vi "Streamlined FPGA.vi"() -> ()   [LabVIEW 2009]
uses:
  <vilib>/eio/EIONode/EIONode.xnode
  <vilib>/rvi/eio/nirviEIOImplementation/nirviEIOImplementation.xnode
  <vilib>/rvi/eio/common/nirviEmuTemplateMethod_noerrors.vi
  <vilib>/rvi/eio/common/nirviEmuClasses.ctl
  Instance           3 24Saved   Streamlined FPGA .vi
  Instance           4 24Saved   Streamlined FPGA .vi
  Instance           5 24Saved   Streamlined FPGA .vi
  Instance           2 24Saved   Streamlined FPGA .vi
  <vilib>/rvi/DataTransferAndStorage/Container/XNode/niFpgaContainer.xnode
  <vilib>/rvi/interface/RandomDataEmulation/niFpgaRandomDataHandleErrors.vi
  <vilib>/rvi/interface/RandomDataEmulation/nirviRandomDataFPGAFIFO.vi
  <vilib>/rvi/DataTransferAndStorage/Container/Common/niFpgaContainerMethod.ctl
  <vilib>/rvi/DataTransferAndStorage/Container/Common/niFpgaTransferTypeControl.ctl
panel:
  in  "smooth":bool
  out ">= x":bool
  out ">= y":bool
  out "xmax":i32
  out "xval":i32
  out "xmin":i32
  out ">=":bool
  in  "Rec2 Ymin":i32
  in  "Rec2 Xmin":i32
  in  "Rec1 Ymin":i32
  in  "Rec1 Xmin":i32
  in  "Rec2 Ymax":i32
  in  "Rec1 Ymax":i32
  in  "Rec2 Xmax":i32
  in  "Rec1 Xmax":i32
  out "sort!":bool
  in  "Maximum Width":i16
  in  "Maximum Height":i16
  in  "trigger on all":bool
  out "sort pulse":i16
  in  "Baselines":i16[](array[numeric])=[0, 0, 0, 0]
  in  "Sb":i8(ring)=1 items=["PMT1", "PMT2", "PMT3", "PMT4"]
  in  "Sa":i8(ring) items=["PMT1", "PMT2", "PMT3", "PMT4"]
  in  "Sort Case":i8(ring)=1 items=["FP", "Magnitude"]
  out "Full 2":bool
  in  "sort?":bool
  out "Drop counter":u32
  out "sort counter":u32
  in  "PMT to detect drops on":u8
  in  "Minimum Height":i16
  in  "Minimum Width":i16
  in  "Ticks between acquires (Ticks)":u32=200
  in  "Gain 1":i16(slide) scale=-32767.0..32767.0
  in  "Gain 2":i16(slide) scale=-32767.0..32767.0
  in  "Gain 3":i16(slide) scale=-32767.0..32767.0
  in  "Gain 4":i16(slide) scale=-32767.0..32767.0
  in  "amplitude":i16
  in  "1/Frequency \n(ticks)":u32
  in  "Burst \nCycles":i32
  in  "delay [us]":u32=20 min=1 max=8000
  # "Acquisition and Detection"
  # "FP and Sorting Parameters"
  # "Sorting Pulse\nGenerator"
  # "Events"
  # "PMT Controls"
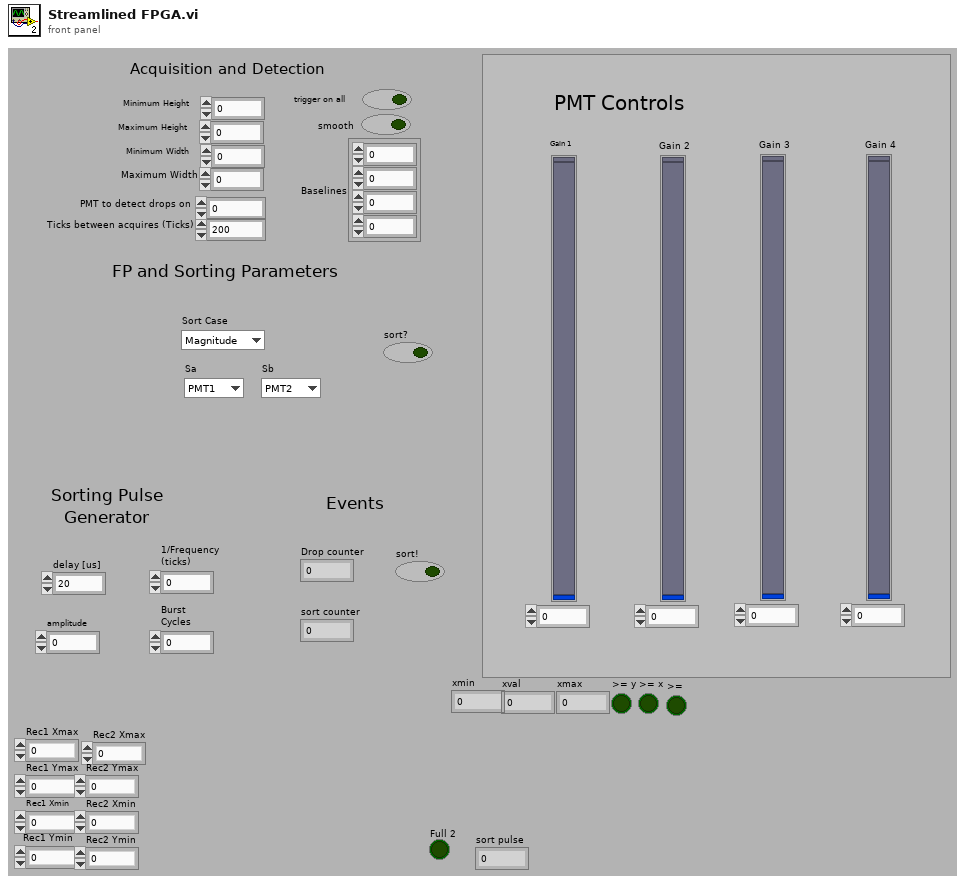
[diagram p1: front panel]
types:
  T1 = typedef "nirviEmuClasses.ctl" = enum16{"IO Read", "IO Write", "Method", "Property Read", "Property Write"}
  T2 = typedef "niFpgaContainerMethod.ctl" = enum16{"Write", "Read", "Clear", "Get Number of Elements to Write", "Get Number of Elements to Read", "Enable", "Disable", "Flush and Disable", "Get Stream State"}
  T3 = typedef "niFpgaTransferTypeControl.ctl" = enum16{"Target-Scoped", "Host to Target - DMA", "Target to Host - DMA", "Peer to Peer Reader", "Peer to Peer Writer", "Bidirectional"}
  T4 = cluster{"Rec1 Xmax":i32, "Rec1 Ymax":i32, "Rec1 Xmin":i32, "Rec1 Ymin":i32, "Rec2 Xmax":i32, "Rec2 Ymax":i32, "Rec2 Xmin":i32, "Rec2 Ymin":i32}
  T5 = cluster{bool, "max":i16[], "sum":i32[], "time inside":i32, "time outside":i32, "timeoutside-1":i32}
  T6 = cluster{"maxes":i16[], "sums":i32[], "time inside":i32, "time outside":i32}
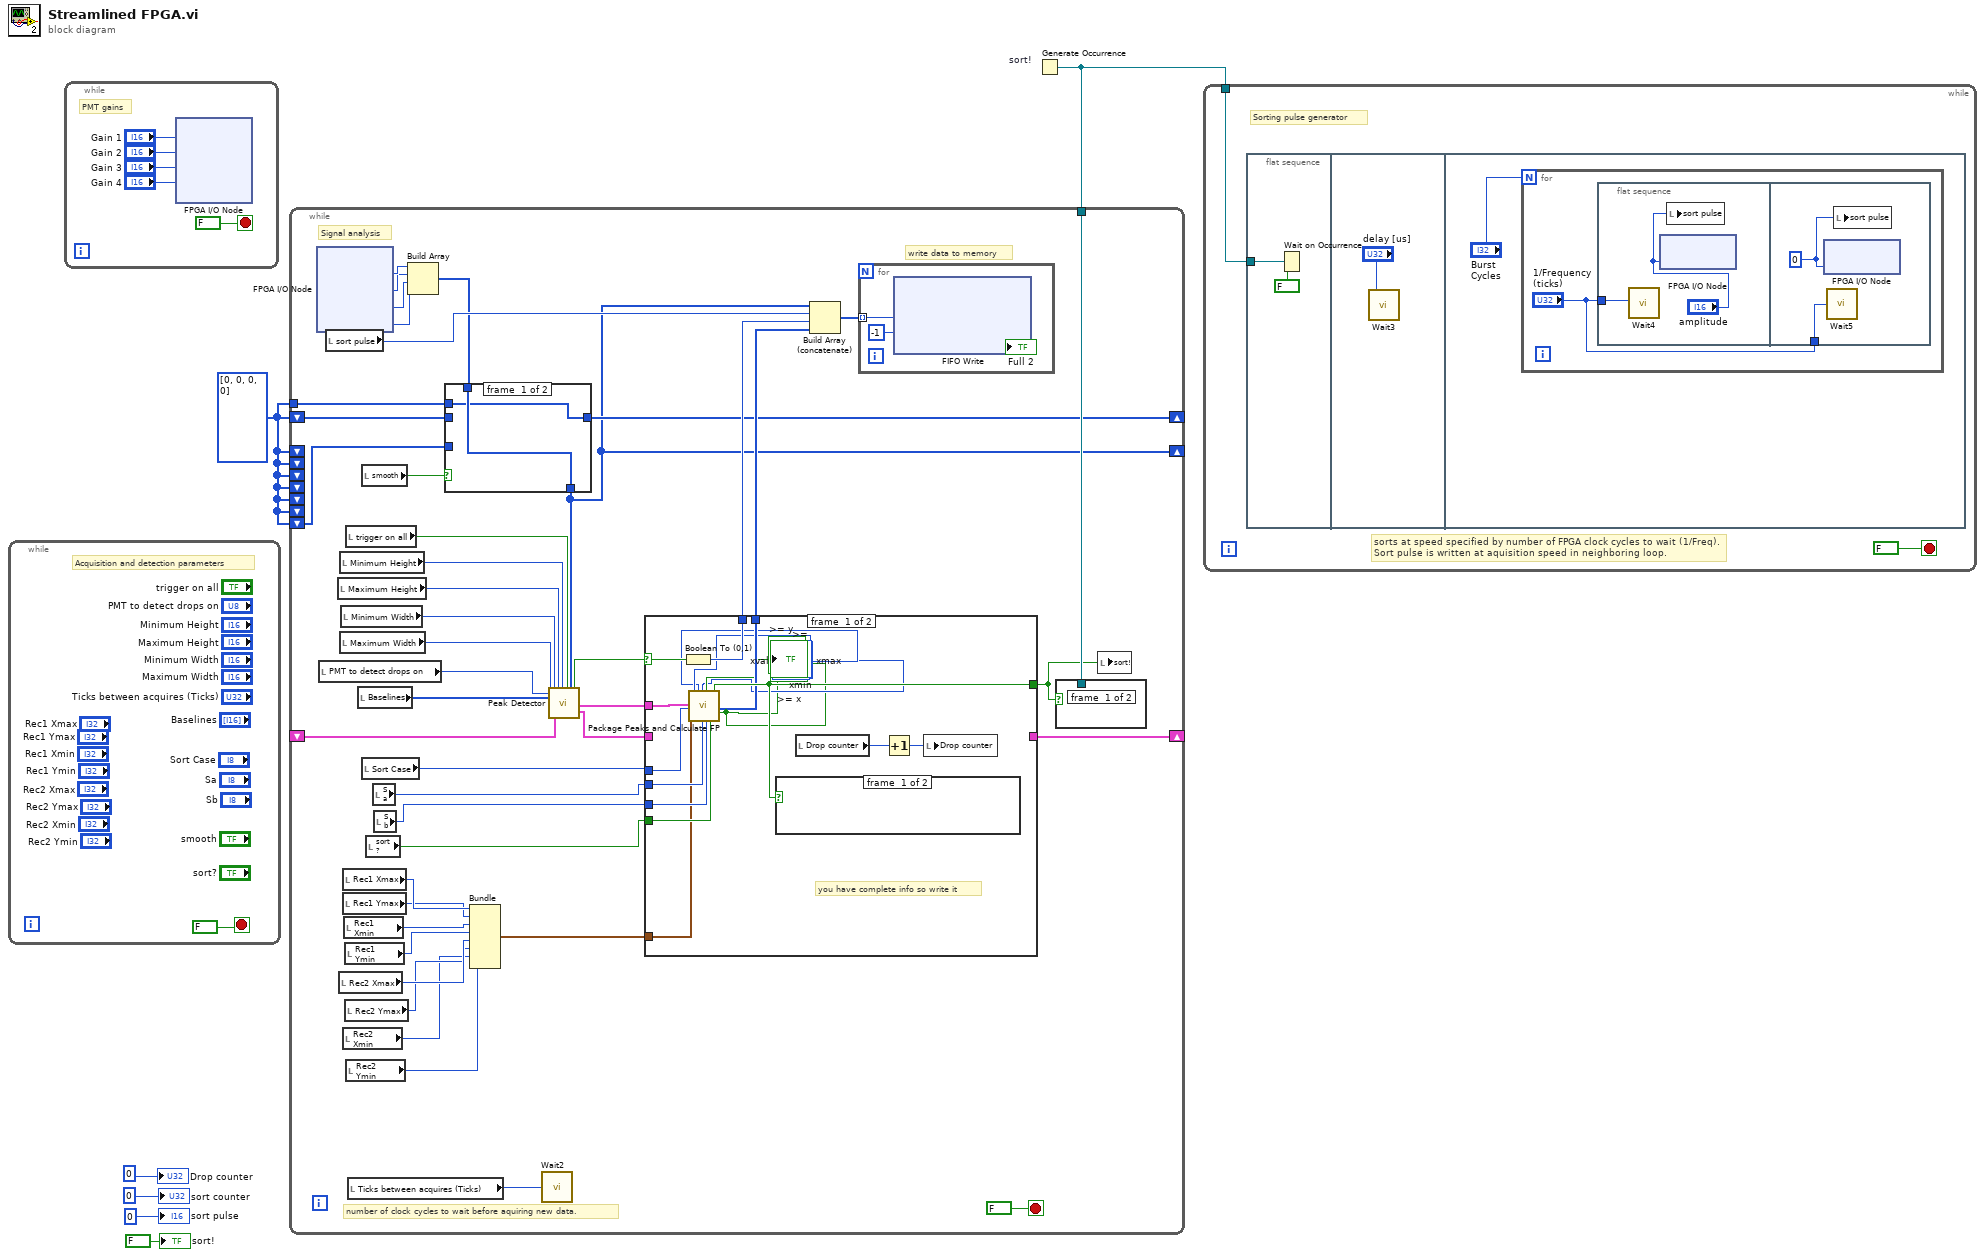
[diagram p0: block diagram]
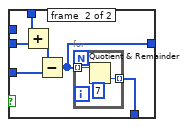
[diagram p2: hidden frame]
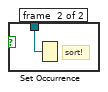
[diagram p3: hidden frame]
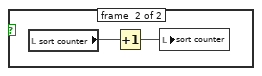
[diagram p4: hidden frame]
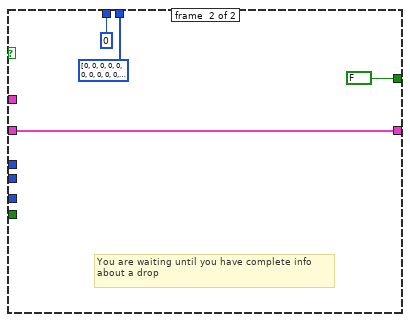
[diagram p5: hidden frame]
diagram:
  w1 = i32[] [0, 0, 0, 0] ("appended array")
  n1 = while {
    stop <- FALSE stop-if-true
    # "Acquisition and detection parameters"
  }
  n2 = while {
    stop <- FALSE stop-if-true
    # "PMT gains"
    n3 = xnode "FPGA I/O Node"("AO0"="Gain 1", "AO1"="Gain 2", "AO2"="Gain 3", "AO3"="Gain 4") -> ()  [unwired: 4 in, 4 out]
  }
  n4 = Generate Occurrence "sort!"() -> (w6:refnum<k4>)
  n5 = while {
    shift-right: [w99] -> _
    shift-left: _ -> [w86]
    tunnel: w6 -> [w84]
    shift-right: [w59] -> _
    shift-left: w1 -> [w63]
    shift-right: [w58] -> _
    shift-left: w1 -> [_]
    shift-left: w1 -> [_]
    shift-left: w1 -> [_]
    shift-left: w1 -> [_]
    shift-left: w1 -> [_]
    shift-left: w1 -> [_]
    shift-left: w1 -> [w62]
    tunnel: w1 -> [w61]
    stop <- FALSE stop-if-true
    # "number of clock cycles to wait before aquiring new data."
    # "Signal analysis"
    # "write data to memory"
    n6 = xnode "FPGA I/O Node"() -> ("AI0"=w98:i16, "AI1"=w97:i16, "AI2"=w96:i16, "AI3"=w95:i16)  [unwired: 4 in, 4 out]
    n7 = local read "PMT to detect drops on"() -> (w76:u8)
    n8 = local read "sort pulse"() -> (w83:i16)
    n9 = local read "Maximum Height"() -> (w79:i16)
    n10 = local read "Rec2 Xmax"() -> (w68:i32)
    n11 = local read "Minimum Height"() -> (w80:i16)
    n12 = local read "Maximum Width"() -> (w77:i16)
    n13 = local read "Minimum Width"() -> (w78:i16)
    n14 = local read "Rec1 Xmax"() -> (w72:i32)
    n15 = local read "Rec1 Ymax"() -> (w71:i32)
    n16 = local read "Rec2 Xmin"() -> (w66:i32)
    n17 = local read "Rec1 Xmin"() -> (w70:i32)
    n18 = local read "Rec1 Ymin"() -> (w69:i32)
    n19 = local read "Rec2 Ymax"() -> (w67:i32)
    n20 = local read "trigger on all"() -> (w85:bool)
    n21 = local read "Rec2 Ymin"() -> (w65:i32)
    n22 = local read "Ticks between acquires (Ticks)"() -> (w94:u32)
    n23 = local read "Baselines"() -> (w75:i16[])
    n24 = local read "smooth"() -> (w57:bool)
    n25 = local read "Sort Case"() -> (w93:i8)
    n26 = local read "sort?"() -> (w90:bool)
    n27 = local read "Sa"() -> (w92:i8)
    n28 = local read "Sb"() -> (w91:i8)
    n29 = Build Array(w98, w97, w96, w95) -> (w60:i16[])
    n30 = case shown="True" w57 {
      tunnel: [w101 w103] -> w59
      tunnel: w62 -> [_ w108]
      tunnel: w63 -> [_ w107]
      tunnel: w60 -> [w102 w106]
      tunnel: [w102 w105] -> w58
      tunnel: w61 -> [w101 _]
      frame #0 {
      }
      frame #1 {
        n31 = Add(x=w106, y=w107) -> (x+y=w104:i32[])
        n32 = Subtract(x=w104, y=w108) -> (x-y=w103:i32[])
        n33 = for {
          tunnel: [w110] -> w105 mode=indexing
          tunnel: w103 -> [w109] mode=indexing
          n34 = Quotient & Remainder(x=w109, y=7 ("AI3")) -> (floor(x/y)=w110:i32)  [unwired: 1 out]
        }
      }
    }
    n35 = Bundle("Rec1 Xmax"=w72, "Rec1 Ymax"=w71, "Rec1 Xmin"=w70, "Rec1 Ymin"=w69, "Rec2 Xmax"=w68, "Rec2 Ymax"=w67, "Rec2 Xmin"=w66, "Rec2 Ymin"=w65) -> (w64:T4)  [unwired: 1 in]
    n36 = call "Wait2"("Count(Ticks)"=w94) -> ()  [unwired: 1 out]
    n37 = call "Peak Detector.vi"("Maximum Width"=w77, "PMT to trigger on (0,1,2,3)"=w76, "Baselines"=w75, "Minimum Width"=w78, "shifts in"=w86, "Maximum Height"=w79, "Minimum Height"=w80, "trigger on all"=w85, "s1,s2,s3,s4"=w58) -> ("peak complete?"=w89:bool, "shifts out"=w87:T5, "peaks data"=w88:T6)  [unwired: 16 in]
    n38 = case shown="True" w89 {
      selector: w89 -> [w227 _]
      tunnel: [_ w238] -> w99
      tunnel: [w225 FALSE ("sort!")] -> w74
      tunnel: w93 -> [w223 _]
      tunnel: w92 -> [w231 _]
      tunnel: w91 -> [w230 _]
      tunnel: w90 -> [w229 _]
      tunnel: w87 -> [_ w238]
      tunnel: w88 -> [w228 _]
      tunnel: [w226 i16 0] -> w81
      tunnel: [w224 i32[] [0, 0, 0, 0, 0, 0, 0, 0, 0, 0, 0, 0] ("M1,M2,M3,M4,S1,S2,S3,S4,Tin,Tout,FP")] -> w73
      tunnel: w64 -> [w222 _]
      frame #0 {
        # "you have complete info so write it"
        n39 = Boolean To (0,1)(Boolean=w227) -> (0, 1=w226:i16)
        n40 = call "Package Peaks and Calculate FP.vi"("peaks data"=w228, "Sort Case"=w223, "Rectangle Positions"=w222, "Sa"=w231, "Sb"=w230, "sort?"=w229) -> ("xmin"=→"xmin":i32, "xval"=→"xval":i32, "xmax"=→"xmax":i32, ">="=→">=":bool, "sort!"=w225:bool, "M1,M2,M3,M4,S1,S2,S3,S4,Tin,Tout,FP,Sort?"=w224:i32[], ">= y"=→">= y" →">= x":bool)  [unwired: 14 in, 1 out]
        n41 = case shown="True" w225 {
          frame #0 {
          }
          frame #1 {
            n42 = local read "sort counter"() -> (w235:u32)
            n43 = Increment(x=w235) -> (x+1=w234:u32)
            n44 = local write "sort counter"(w234) -> ()
          }
        }
        n45 = local read "Drop counter"() -> (w233:u32)
        n46 = Increment(x=w233) -> (x+1=w232:u32)
        n47 = local write "Drop counter"(w232) -> ()
      }
      frame #1 {
        # "You are waiting until you have complete info about a drop"
      }
    }
    n48 = Build Array (concatenate)(w58, w83, w81, w73) -> (w82:i32[])
    n49 = for {
      tunnel: w82 -> [w115] mode=indexing
      n50 = xnode ("FIFO Write")("Element"=w115, "Timeout"=-1) -> ("Timed Out?"=→"Full 2":bool)  [unwired: 1 in, 1 out]
    }
    n51 = case shown="True" w74 {
      tunnel: w84 -> [_ w112]
      frame #0 {
      }
      frame #1 {
        # "sort!"
        n52 = Set Occurrence(w112) -> ()
      }
    }
    n53 = local write "sort!"(w74) -> ()
  }
  n54 = while {
    tunnel: w6 -> [w240]
    stop <- FALSE stop-if-true
    # "sorts at speed specified by number of FPGA clock cycles to wait (1/Freq).\nSort pulse is written at aquisition speed in neighboring loop."
    # "Sorting pulse generator"
    n55 = flat-sequence {
      tunnel: w240 -> [w242]
      frame #0 {
        n56 = Wait on Occurrence(1:FALSE ("ignore previous (T)"), 2:w242) -> ()  [unwired: 1 in, 1 out]
      }
      frame #1 {
        n57 = call "Wait3"("Count(uSec)"="delay [us]") -> ()  [unwired: 1 out]
      }
      frame #2 {
        n58 = for {
          N: "Burst \nCycles" -> [_]
          n59 = flat-sequence {
            tunnel: "1/Frequency \n(ticks)" -> [w248]
            tunnel: "1/Frequency \n(ticks)" -> [w261]
            frame #0 {
              n60 = call "Wait4"("Count(Ticks)"=w248) -> ()  [unwired: 1 out]
              n61 = xnode "FPGA I/O Node"("AO4"="amplitude") -> ()  [unwired: 1 in, 1 out]
              n62 = local write "sort pulse"("amplitude") -> ()
            }
            frame #1 {
              w260 = i16 0 ("sort pulse")
              n63 = xnode "FPGA I/O Node"("AO4"=w260) -> ()  [unwired: 1 in, 1 out]
              n64 = call "Wait5"("Count(Ticks)"=w261) -> ()  [unwired: 1 out]
              n65 = local write "sort pulse"(w260) -> ()
            }
          }
        }
      }
    }
  }
  "sort counter" <- u32 0 ("event counter")
  "Drop counter" <- u32 0 ("Drop counter")
  "sort pulse" <- i16 0 ("event counter")
  "sort!" <- FALSE ("sort!")
